vi "Peregrine_open_serial.vi"() -> ()   [LabVIEW 2019]
uses:
  <vilib>/Instr/_visa.llb/VISA Configure Serial Port (Instr).vi
panel:
  out "Speed":i16
  out "Position":i32
  out "Command":i32
  out "Address":u8
  out "Closed loop":bool
  out "Fdir":bool
  out "Limit -":bool
  out "Limit +":bool
  out "Emg stop":bool
  out "Running":bool
  out "Boolean array":bool[](array[boolean])
  out "Status message from peregrine":string
  in  "COM Port for serial\nconnection. Check device\nmanager.":string
  # "VI for checking status from peregrine board"
  # "Decoded status message \nfrom peregrine"
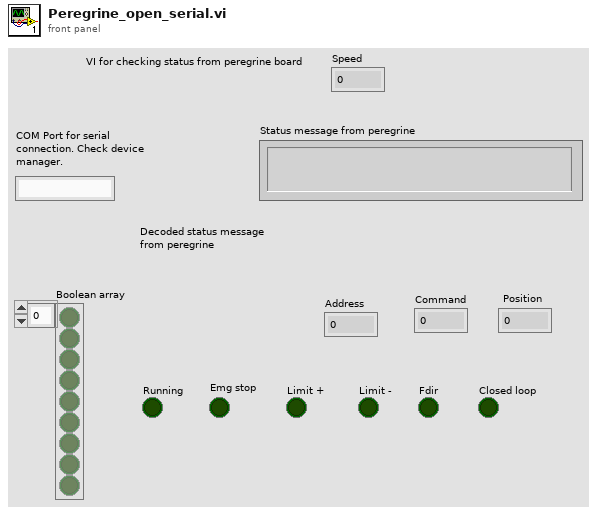
[diagram p1: front panel]
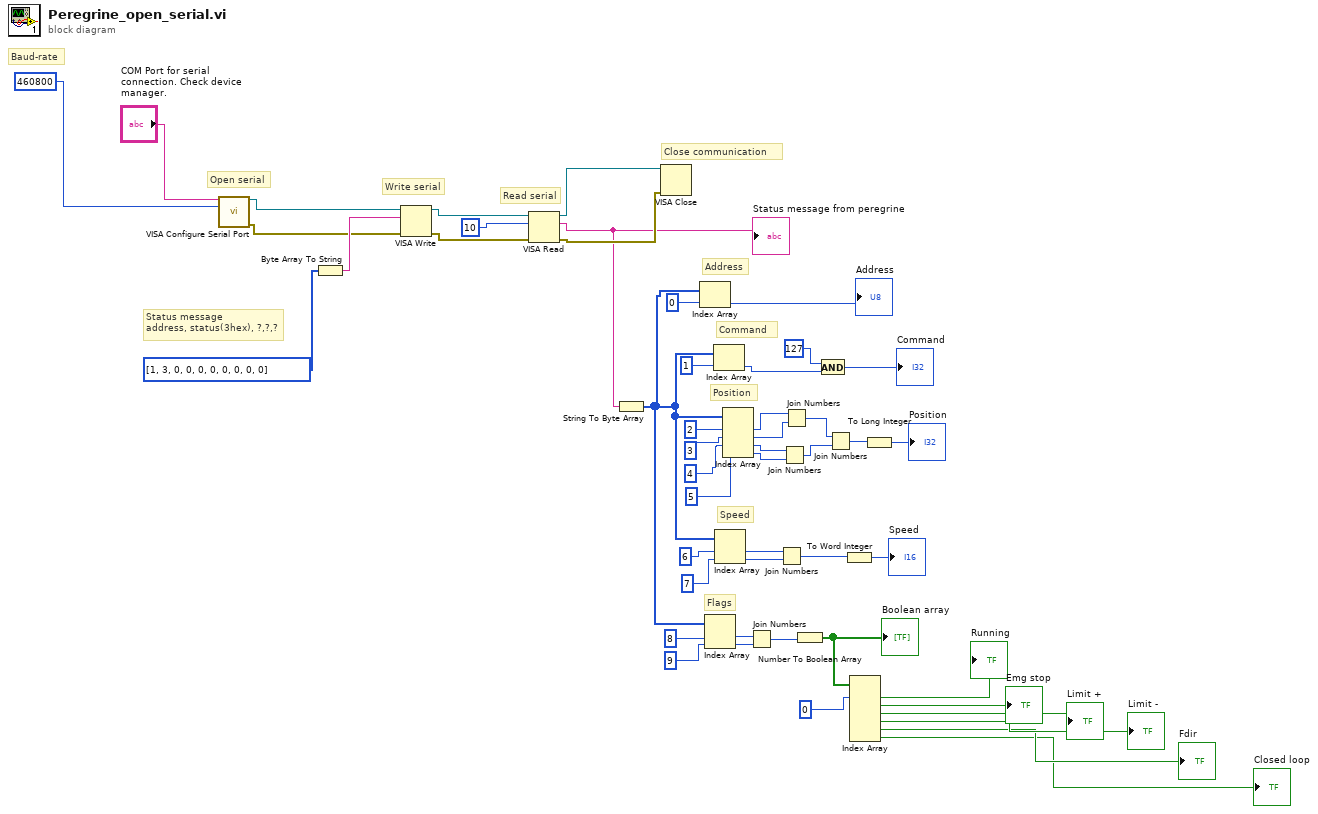
[diagram p0: block diagram]
diagram:
  # "Command"
  # "Address"
  # "Flags"
  # "Speed"
  # "Position"
  # "Close communication"
  # "Read serial"
  # "Write serial"
  # "Open serial"
  # "Status message\naddress, status(3hex), ?,?,?"
  # "Baud-rate"
  n1 = call-poly "VISA Configure Serial Port"("VISA resource name"="COM Port for serial\nconnection. Check device\nmanager.", "baud rate (9600)"=460800) -> ("VISA resource name out"=w48:refnum<visa-resource-name>, "error out"=w41:errorcluster)  [unwired: 12 in]
  n2 = Byte Array To String(unsigned byte array=i8[] [1, 3, 0, 0, 0, 0, 0, 0, 0, 0]) -> (string=w46:string)
  n3 = VISA Write(VISA resource name=w48, write buffer=w46, error in (no error)=w41) -> (VISA resource name out=w44:refnum<visa-resource-name>, error out=w45:errorcluster)  [unwired: 1 out]
  n4 = VISA Read(VISA resource name=w44, byte count=10, error in (no error)=w45) -> (VISA resource name out=w42:refnum<visa-resource-name>, read buffer=w39:string, error out=w40:errorcluster)  [unwired: 1 out]
  "Status message from peregrine" <- w39
  n5 = String To Byte Array(string=w39) -> (unsigned byte array=w31:u8[])
  n6 = VISA Close(VISA resource name=w42, error in (no error)=w40) -> ()  [unwired: 1 out]
  n7 = Index Array(array=w31, index=0) -> (element=→"Address":u8)
  n8 = Index Array(array=w31, index #1=8, index #2=9) -> (element #1=w21:u8, element #2=w20:u8)
  n9 = Index Array(array=w31, index=1) -> (element=w23:u8)
  n10 = Index Array(array=w31, index #1=6, index #2=7) -> (element #1=w7:u8, element #2=w6:u8)
  n11 = Index Array(array=w31, index #1=2, index #2=3, index #3=4, index #4=5) -> (element #1=w29:u8, element #2=w28:u8, element #3=w27:u8, element #4=w26:u8)
  n12 = Join Numbers(hi=w21, lo=w20) -> ((hi.lo)=w18:u16)
  n13 = Join Numbers(hi=w7, lo=w6) -> ((hi.lo)=w5:u16)
  n14 = Join Numbers(hi=w27, lo=w26) -> ((hi.lo)=w25:u16)
  n15 = Join Numbers(hi=w29, lo=w28) -> ((hi.lo)=w24:u16)
  n16 = Number To Boolean Array(number=w18) -> (Boolean array=w16:bool[])
  "Boolean array" <- w16
  n17 = And(x=127, y=w23) -> (x .and. y?=→"Command":i32)
  n18 = Join Numbers(hi=w24, lo=w25) -> ((hi.lo)=w19:u32)
  n19 = To Word Integer(number=w5) -> (16bit integer=→"Speed":i16)
  n20 = Index Array(array=w16, index #1=0) -> (element #1=→"Running":bool, element #2=→"Emg stop":bool, element #3=→"Limit +":bool, element #4=→"Limit -":bool, element #5=→"Fdir":bool, element #6=→"Closed loop":bool)  [unwired: 5 in]
  n21 = To Long Integer(number=w19) -> (32bit integer=→"Position":i32)
